vi "TextfiletoRPM.vi"(10 "Tyre Diameter(m)":sgl=0.5, 11 "file path (dialog if empty)":path=path "C:/Users/arda/Desktop/Thesis/random.txt") -> (2 "Array":dbl[](array[numeric])=[0.0, 0.0, 0.0, 0.0, 0.0, 0.0, 0.0, 0.0, 0.0, 0.0, 0.0, 0.0, 0.03536776304244995, 0.30062598586082456, 0.9549296021461487, 1.7507042706012725, 2.3165884792804716, 2.9885759770870206, 3.83740229010582, 4.597809195518494, 4.863067418336868, 4.969170707464218, 5.0045384705066684, 5.092957878112793, 5.146009522676468, 5.446635508537293, 5.641158205270767, 6.0302035987377165, 6.472300636768341, 6.914397674798965, 7.303443068265914, 7.515649646520615, 7.657120698690414, 7.7632239878177645, 7.851643395423889, 7.869327276945114, 7.81627563238144, 7.551017409563065, 7.055868726968765, 6.543036162853241, 6.118623006343841, 5.711893731355667, 5.128325641155243, 4.438654261827469, 3.9258216977119447, 3.6959312379360196, 3.6075118303298948, 3.4483568966388702, 3.2538341999053952, 3.1477309107780456, 3.1477309107780456, 3.0769953846931455, 2.7763693988323213, 2.3165884792804716, 2.139749664068222, 2.122065782546997, 2.122065782546997, 2.122065782546997, 2.175117427110672, 2.2281690716743467, 2.5995305836200715, 2.705633872747421, 2.8117371618747713, 2.864788806438446, 3.023943740129471, 3.1477309107780456, 3.200782555341721, 3.2538341999053952, 3.58982794880867, 4.102660512924194, 4.6862286031246185, 5.269796693325043, 5.764945375919342, 6.083255243301392, 6.277777940034866, 6.436932873725891, 6.613771688938141, 6.808294385671616, 6.949765437841415, 6.985133200883865, 6.8967137932777405, 6.808294385671616, 6.596087807416915, 6.543036162853241, 6.489984518289567, 6.348513466119766, 6.242410176992416, 6.118623006343841, 6.047887480258942, 5.641158205270767, 4.827699655294419, 3.8904539346694946, 3.006259858608246, 2.5111111760139466, 2.122065782546997, 1.6092332184314728, 1.0256651282310485, 0.6366197347640992, 0.3890453934669495, 0.0, 0.0, 0.0, 0.0, 0.0, 0.0, 0.0, 0.0, 0.0, 0.0, 0.0, 0.0, 0.0, 0.0, 0.0, 0.0, 0.0, 0.0, 0.0, 0.0, 0.0, 0.0, 0.0, 0.0, 0.0, 0.0, 0.0, 0.0, 0.0, 0.0, 0.0, 0.0, 0.0, 0.0, 0.0, 0.0, 0.0, 0.0, 0.0, 0.03536776304244995, 0.33599374890327455, 1.0787167727947236, 2.0690141379833222, 2.9001565694808957, 3.34225360751152, 3.51909242272377, 3.678247356414795, 4.031924986839295, 4.491705906391144, 4.898435181379318, 5.1636934041976925, 5.269796693325043, 5.199061167240143, 4.810015773773193, 3.9965572237968447, 3.0593115031719207, 2.3519562423229217, 2.122065782546997, 2.2281690716743467, 2.4934272944927214, 3.041627621650696, 3.5544601857662204, 4.1380282759666445, 4.509389787912369, 4.880751299858093, 5.216745048761368, 5.499687153100967, 5.676525968313217, 5.871048665046692, 6.224726295471192, 6.5784039258956915, 6.719874978065491, 6.613771688938141, 6.207042413949966, 5.482003271579742, 4.792331892251968, 4.474022024869919, 4.438654261827469, 4.580125313997269, 4.916119062900544, 5.1636934041976925, 5.234428930282593, 5.216745048761368, 5.1636934041976925, 5.0045384705066684, 4.6154930770397185, 4.173396039009094, 3.713615119457245, 3.34225360751152, 3.023943740129471, 2.7763693988323213, 2.5641628205776215, 2.4226917684078217, 2.281220716238022, 2.210485190153122, 2.157433545589447, 2.122065782546997, 2.122065782546997, 2.122065782546997, 2.122065782546997, 2.210485190153122, 2.298904597759247], 3 "time_sp":sgl[](array[numeric])=[0.0, 1.0, 2.0, 3.0, 4.0, 5.0, 6.0, 7.0, 8.0, 9.0, 10.0, 11.0, 12.0, 13.0, 14.0, 15.0, 16.0, 17.0, 18.0, 19.0, 20.0, 21.0, 22.0, 23.0, 24.0, 25.0, 26.0, 27.0, 28.0, 29.0, 30.0, 31.0, 32.0, 33.0, 34.0, 35.0, 36.0, 37.0, 38.0, 39.0, 40.0, 41.0, 42.0, 43.0, 44.0, 45.0, 46.0, 47.0, 48.0, 49.0, 50.0, 51.0, 52.0, 53.0, 54.0, 55.0, 56.0, 57.0, 58.0, 59.0, 60.0, 61.0, 62.0, 63.0, 64.0, 65.0, 66.0, 67.0, 68.0, 69.0, 70.0, 71.0, 72.0, 73.0, 74.0, 75.0, 76.0, 77.0, 78.0, 79.0, 80.0, 81.0, 82.0, 83.0, 84.0, 85.0, 86.0, 87.0, 88.0, 89.0, 90.0, 91.0, 92.0, 93.0, 94.0, 95.0, 96.0, 97.0, 98.0, 99.0, 100.0, 101.0, 102.0, 103.0, 104.0, 105.0, 106.0, 107.0, 108.0, 109.0, 110.0, 111.0, 112.0, 113.0, 114.0, 115.0, 116.0, 117.0, 118.0, 119.0, 120.0, 121.0, 122.0, 123.0, 124.0, 125.0, 126.0, 127.0, 128.0, 129.0, 130.0, 131.0, 132.0, 133.0, 134.0, 135.0, 136.0, 137.0, 138.0, 139.0, 140.0, 141.0, 142.0, 143.0, 144.0, 145.0, 146.0, 147.0, 148.0, 149.0, 150.0, 151.0, 152.0, 153.0, 154.0, 155.0, 156.0, 157.0, 158.0, 159.0, 160.0, 161.0, 162.0, 163.0, 164.0, 165.0, 166.0, 167.0, 168.0, 169.0, 170.0, 171.0, 172.0, 173.0, 174.0, 175.0, 176.0, 177.0, 178.0, 179.0, 180.0, 181.0, 182.0, 183.0, 184.0, 185.0, 186.0, 187.0, 188.0, 189.0, 190.0, 191.0, 192.0, 193.0, 194.0, 195.0, 196.0, 197.0, 198.0, 199.0, 200.0])   [LabVIEW 2016]
uses:
  <vilib>/Utility/file.llb/Read Delimited Spreadsheet (DBL).vi
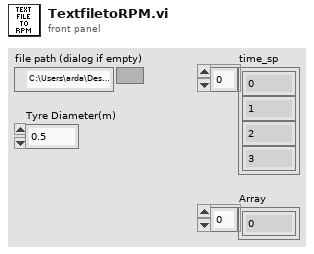
[diagram p1: front panel]
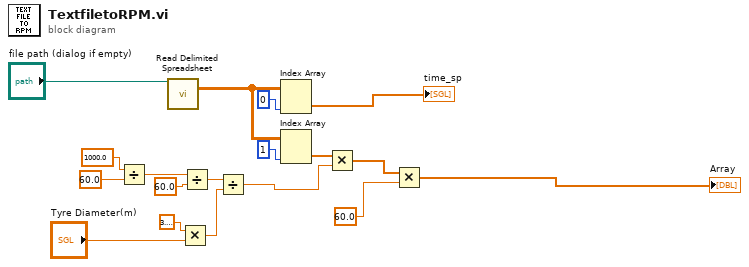
[diagram p0: block diagram]
diagram:
  n1 = Divide(x=sgl 1000.0, y=sgl 60.0) -> (x/y=w16:sgl)
  n2 = call-poly <vilib>:"Read Delimited Spreadsheet.vi"("file path (dialog if empty)"="file path (dialog if empty)") -> ("all rows"=w7:dbl[][])  [unwired: 9 in, 5 out]
  n3 = Multiply(x=sgl 3.1415927, y="Tyre Diameter(m)") -> (x*y=w14:sgl)
  n4 = Divide(x=w16, y=sgl 60.0) -> (x/y=w18:sgl)
  n5 = Divide(x=w18, y=w14) -> (x/y=w5:sgl)
  n6 = Index Array(array=w7, index (col)=0 ("index (row)")) -> (element=→"time_sp":dbl[])  [unwired: 1 in]
  n7 = Index Array(array=w7, index (col)=1 ("index (row)")) -> (element=w1:dbl[])  [unwired: 1 in]
  n8 = Multiply(x=w1, y=w5) -> (x*y=w4:dbl[])
  n9 = Multiply(x=w4, y=sgl 60.0) -> (x*y=→"Array":dbl[])
